vi "Replace Substring.vi"(4 "mode (literal)":enum16{"literal", "wild card", "reg expr"}(ring), 6 "match whole word (F)":bool, 7 "replace all (T)":bool=TRUE, 8 "case matching (sensitive)":T1=enum."system", 9 "replacement":string, 10 "pattern":string, 11 "text":string) -> (1 "# replacements":i32, 3 "text out":string)   [LabVIEW 2015, in "TLB` Template.lvlib" / "Tools_String.lvlib"]
doc: "Replaces 1 or all instences of a pattern in a string.\nMode determines the match criteria: a literal string, a literal string with wildcards or a regular expression.\n\nmatch whole words is currently ignored\ncase insensitive regular expressions don't quite work yetTLB Prime - Application Template 1.3.0.24\nNorm Kirchner, NI Systems Engineering - NI\nCopyright (c) 2014, NI"
uses:
  Tools_String.lvlib
  <vilib>/FTP/util/Case Matching.ctl
  <vilib>/FTP/NI_FTP.lvlib
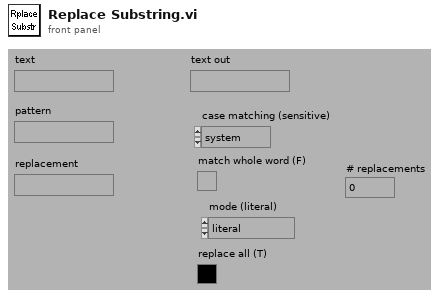
[diagram p1: front panel]
types:
  T1 = typedef "NI_FTP.lvlib/Case Matching.ctl" = enum16{"a != A", "a == A", "system"}
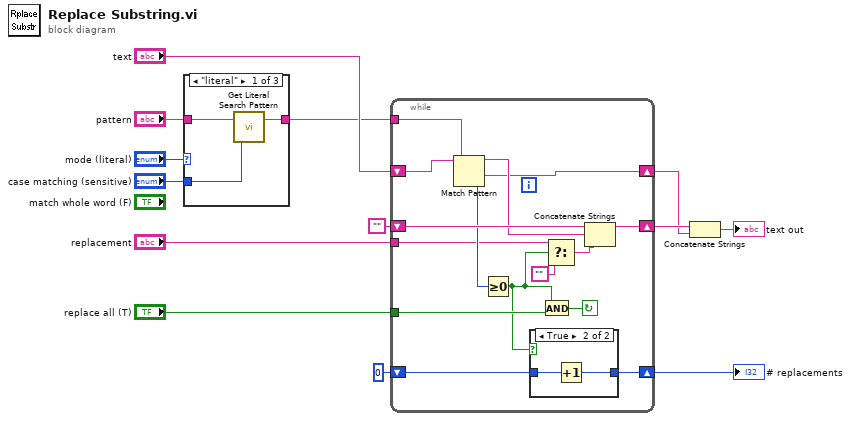
[diagram p0: block diagram]
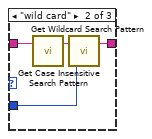
[diagram p3: hidden frame]
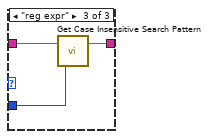
[diagram p4: hidden frame]
diagram:
  n1 = case shown="\"literal\"" "mode (literal)" {
    tunnel: "pattern" -> [w16 w20 w23]
    tunnel: [w15 w18 w22] -> w8
    tunnel: "case matching (sensitive)" -> [w14 w17 w21]
    frame "literal" {
      n2 = call "Get Literal Search Pattern.vi"("case matching (sensitive)"=w14, "literal string"=w16) -> ("regular expression"=w15:string)  [unwired: 1 out]
    }
    frame "wild card" {
      n3 = call "Get Wildcard Search Pattern.vi"("literal string"=w20) -> ("regular expression"=w19:string)  [unwired: 1 in, 1 out]
      n4 = call "Get Case Insensitive Search Pattern.vi"("case matching (sensitive)"=w17, "regular expression"=w19) -> ("case insensitive regular expression"=w18:string)  [unwired: 1 out]
    }
    frame "reg expr" {
      n5 = call "Get Case Insensitive Search Pattern.vi"("case matching (sensitive)"=w21, "regular expression"=w23) -> ("case insensitive regular expression"=w22:string)  [unwired: 1 out]
    }
  }
  n6 = while {
    shift-left: 0 -> [w25]
    shift-right: [w24] -> w1
    tunnel: "replace all (T)" -> [w28]
    tunnel: w8 -> [w29]
    shift-left: "text" -> [w31]
    shift-right: [w30] -> w4
    tunnel: "replacement" -> [w34]
    shift-left: "" -> [w38]
    shift-right: [w37] -> w5
    stop <- w27 continue-if-true
    n7 = Match Pattern(string=w31, regular expression=w29) -> (before substring=w36:string, after substring=w30:string, offset past match=w35:i32)  [unwired: 2 out]
    n8 = Greater Or Equal To 0?(x=w35) -> (x >= 0?=w26:bool)
    n9 = case shown="True" w26 {
      tunnel: w25 -> [w39 w41]
      tunnel: [w39 w40] -> w24
      frame False {
      }
      frame True {
        n10 = Increment(x=w41) -> (x+1=w40:i32)
      }
    }
    n11 = And(x=w26, y=w28) -> (x .and. y?=w27:bool)
    n12 = Select(t=w34, s=w26, f="") -> (s? t:f=w33:string)
    n13 = Concatenate Strings(w38, w36, w33) -> (w37:string)
  }
  "# replacements" <- w1
  n14 = Concatenate Strings(w5, w4) -> (→"text out":string)
